vi "Dequeue Message.vi"(8 "error in (no error)":errorcluster, 11 "Message Queue":refnum<queue>) -> (0 "error out":errorcluster, 1 "Message Data":variant, 2 "Message":string, 3 "dup Message Queue":refnum<queue>)   [LabVIEW 2018, in "Message Queue.lvlib"]
doc: "This VI pulls messages off the Message Queue. It has special error handling to account for an error occurring on the last iteration of the Message Handling Loop.\n\nNo Error - normal Dequeue Element operation.\nError - check if it is an error code we wish to ignore. If so, clear the error and perform a normal Dequeue Element. If not, output the error, and put a 'Stop' message on the Message Queue."
uses:
  Message Queue.lvlib
  Message Cluster.ctl
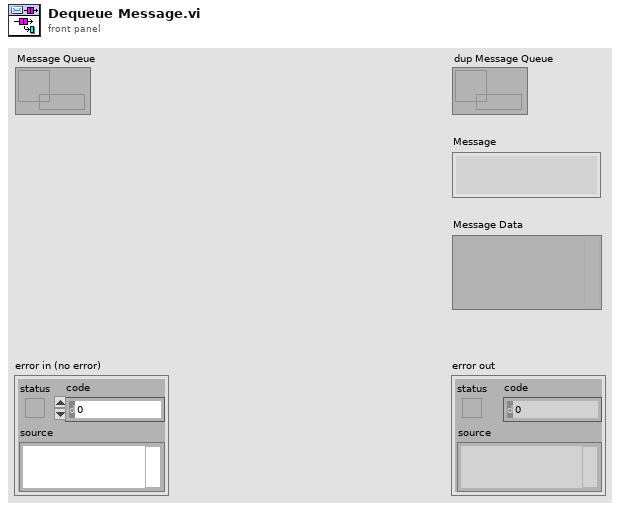
[diagram p1: front panel]
types:
  T1 = typedef "Message Queue.lvlib/Message Cluster.ctl" = cluster{"Message":string, "Message Data":variant}
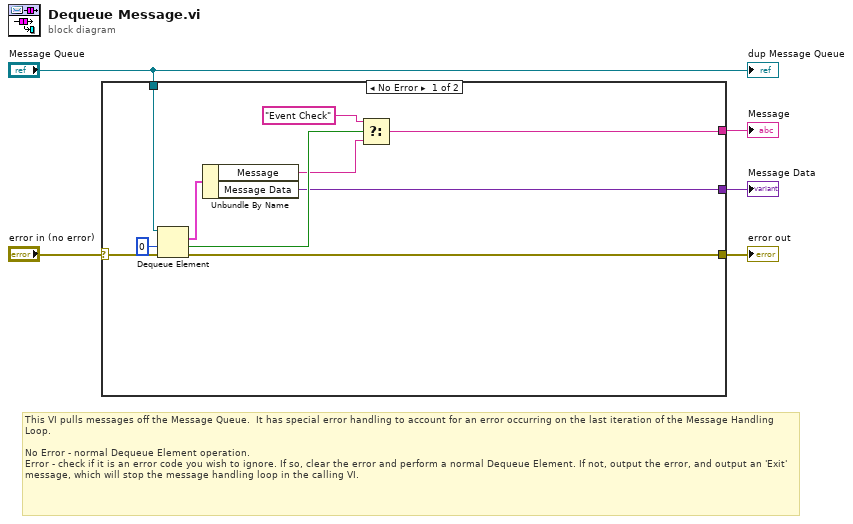
[diagram p0: block diagram]
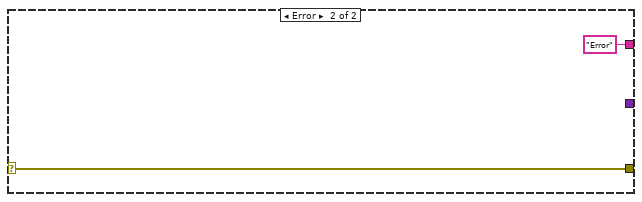
[diagram p2: hidden frame]
diagram:
  # "This VI pulls messages off the Message Queue.  It has special error handling to account for an error occurring on the last iteration of the Message Handling Loop.\n\nNo Error - normal Dequeue Element operation.\nError - check if it is an error code you wish to ignore. If so, clear the error and perform a normal Dequeue Element. If not, output the error, and output an 'Exit' message, which will stop the message handling loop in the calling VI."
  n1 = case shown="No Error" "error in (no error)" {
    selector: "error in (no error)" -> [w15 w16]
    tunnel: "Message Queue" -> [w14 _]
    tunnel: [w12 w16] -> w3
    tunnel: [w9 "Error" ("Message")] -> w2
    tunnel: [w7 _] -> w1
    frame No Error {
      n2 = Dequeue Element(queue=w14, timeout in ms (-1)=0, error in (no error)=w15) -> (element=w8:T1, timed out?=w11:bool, error out=w12:errorcluster)  [unwired: 1 out]
      n3 = Unbundle By Name(w8) -> ("Message"=w6:string, "Message Data"=w7:variant)
      n4 = Select(t="Event Check", s=w11, f=w6) -> (s? t:f=w9:string)
    }
    frame Error {
    }
  }
  "error out" <- w3
  "Message" <- w2
  "Message Data" <- w1
  "dup Message Queue" <- "Message Queue"
